vi "Transmit Frames.vi"(8 "error in (no error)":errorcluster, 11 "uCAN in":refnum<class "uCAN.lvclass">) -> (0 "error out":errorcluster, 3 "uCAN out":refnum<class "uCAN.lvclass">)   [LabVIEW 2021, in "uCanDriver.lvlib" / "uCAN.lvclass"]
uses:
  uCAN.lvclass
  typedefs/frame.ctl
  uCAN.lvclass/uCAN.ctl
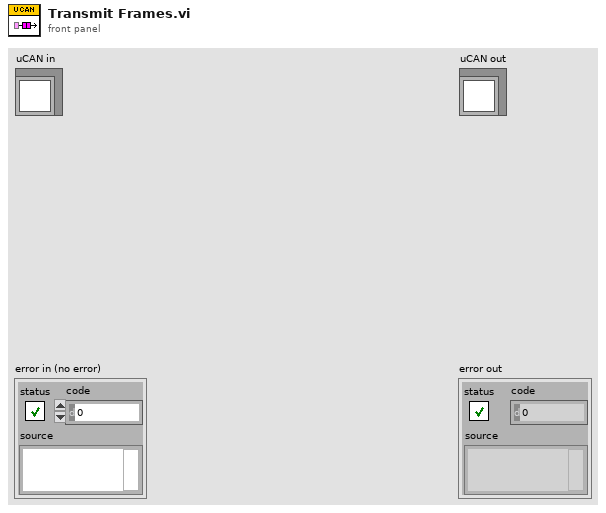
[diagram p1: front panel]
types:
  T1 = typedef "uCanDriver.lvlib/uCAN.lvclass/frame.ctl" = cluster{"Extended":bool, "ID":u32, "Data":u8[], "DLC":u8}
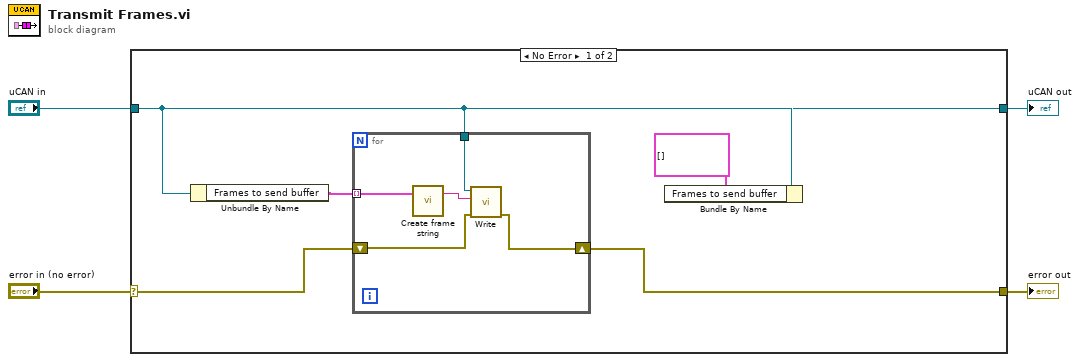
[diagram p0: block diagram]
diagram:
  n1 = case shown="No Error" "error in (no error)" {
    selector: "error in (no error)" -> [w6 w17]
    tunnel: [w5 w17] -> w3
    tunnel: [w8 w16] -> w1
    tunnel: "uCAN in" -> [w9 w16]
    frame No Error {
      n2 = Unbundle By Name(w9) -> ("Frames to send buffer"=w10:T1[])
      n3 = for {
        tunnel: w10 -> [w15] mode=indexing
        tunnel: w9 -> [w13]
        shift-right: [w11] -> w5
        shift-left: w6 -> [w12]
        n4 = call "Create frame string.vi"("Frame"=w15) -> ("String"=w14:string)  [unwired: 2 in]
        n5 = call "Write.vi"("error in (no error)"=w12, "write buffer"=w14, "uCAN in"=w13) -> ("error out"=w11:errorcluster)  [unwired: 8 in]
      }
      n6 = Bundle By Name(cluster=w9, "Frames to send buffer"=T1[] []) -> (w8:refnum<class "uCAN.lvclass">)
    }
    frame Error {
    }
  }
  "error out" <- w3
  "uCAN out" <- w1
